vi "Assemble Default Layout.vi"(9 "Botom View":refnum<class "IViewable.lvclass">, 10 "Left View":refnum<class "IViewable.lvclass">, 11 "Main View":refnum<class "IViewable.lvclass">) -> (3 "ViewManagerDefaultLayout":refnum<class "ViewManagerDefaultLayout.lvclass">)   [LabVIEW 2017, in "ViewManagerDefaultLayout.lvclass"]
uses:
  ViewManagerDefaultLayout.lvclass
  C:/Program Files/National Instruments/LabVIEW 2017/vi.lib/Composed/GPM Packages/mva-framework/Source/Framework/IViewManager/IViewManager/IViewManager.lvclass
  mva-viewable/Source/IViewable/IViewable/IViewable.lvclass
  mva-viewable/Source/IViewManager/IViewManager Messages/Launch Nested Views Msg/Launch Nested Views Msg.lvclass/Launch Nested Views Msg.ctl
  mva-viewable/Source/IViewManager/IViewManager/IViewManager.lvclass/IViewManager.ctl
  mva-viewable/Source/IViewManager/IViewManager Messages/Launch Nested Views Msg/Launch Nested Views Msg.lvclass
  mva-viewable/Source/IViewManager/IViewManager/IViewManager.lvclass
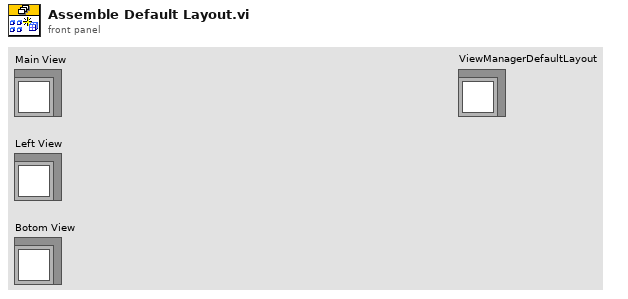
[diagram p1: front panel]
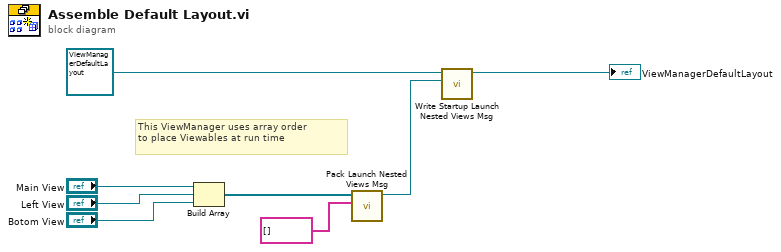
[diagram p0: block diagram]
diagram:
  # "This ViewManager uses array order\nto place Viewables at run time"
  n1 = Build Array("Main View", "Left View", "Botom View") -> (w2:refnum<class "IViewable.lvclass">[])
  n2 = call "Pack Launch Nested Views Msg.vi"("View Labels"=string[] [], "Nested Views"=w2) -> ("Launch Nested Views Msg"=w6:refnum<class "Launch Nested Views Msg.lvclass">)  [unwired: 9 in]
  n3 = call "Write Startup Launch Nested Views Msg.vi"("Launch Nested Views Msg"=w6, "IViewManager in"=refnum<class "ViewManagerDefaultLayout.lvclass"> refnum ("ViewManagerDefaultLayout in")) -> ("IViewManager out"=→"ViewManagerDefaultLayout":refnum<class "ViewManagerDefaultLayout.lvclass">)  [unwired: 9 in]
